vi "startClient.vi"(8 "error in (no error)":errorcluster, 11 "M1M3SAL in":refnum<class "M1M3SAL.lvclass">) -> (0 "error out":errorcluster, 3 "M1M3SAL out":refnum<class "M1M3SAL.lvclass">)   [LabVIEW 2016, in "M1M3SupportCommunicator.lvlib" / "M1M3SAL.lvclass"]
uses:
  M1M3SAL.lvclass
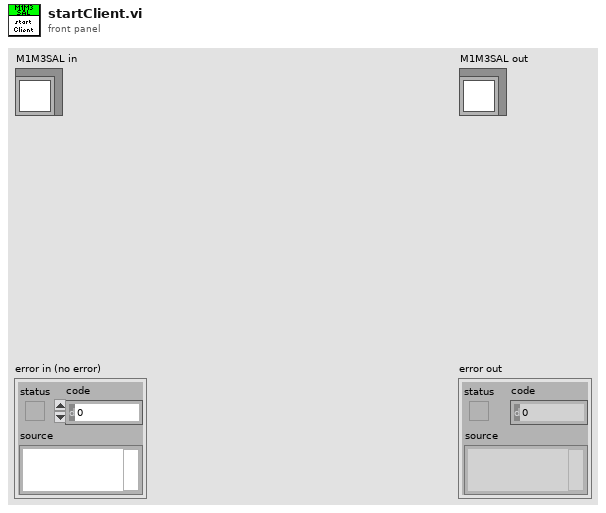
[diagram p1: front panel]
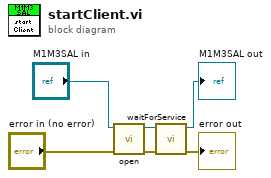
[diagram p0: block diagram]
diagram:
  n1 = call "open.vi"("error in (no error)"="error in (no error)", "M1M3SAL in"="M1M3SAL in") -> ("error out"=w2:errorcluster, "M1M3SAL out"=w5:refnum<class "M1M3SAL.lvclass">)  [unwired: 8 in]
  n2 = call "waitForService.vi"("error in (no error)"=w2, "M1M3SAL in"=w5) -> ("error out"=→"error out":errorcluster, "M1M3SAL out"=→"M1M3SAL out":refnum<class "M1M3SAL.lvclass">)  [unwired: 8 in]
